vi "WaitUntilVIDoneRunning.vi"(8 "error in (no error)":errorcluster, 11 "UI_Interaction_Manager in":refnum<class "UI_Interaction_Manager.lvclass">) -> (0 "error out":errorcluster, 3 "UI_Interaction_Manager out":refnum<class "UI_Interaction_Manager.lvclass">)   [LabVIEW 2011, in "UI_Interaction_Manager.lvclass"]
uses:
  UI_Interaction_Manager.lvclass
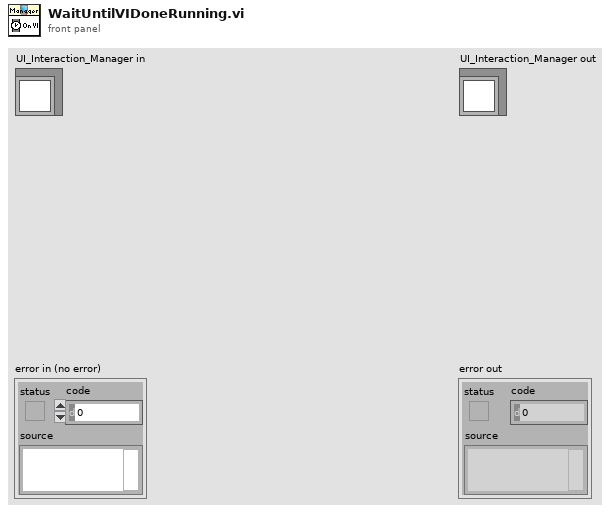
[diagram p1: front panel]
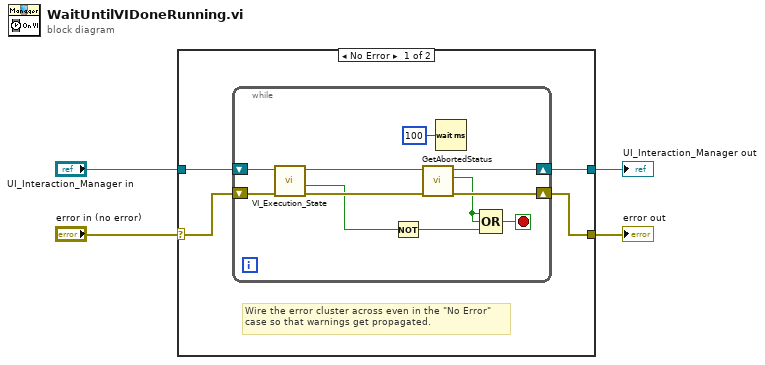
[diagram p0: block diagram]
diagram:
  n1 = case shown="No Error" "error in (no error)" {
    selector: "error in (no error)" -> [w8 w21]
    tunnel: [w7 w21] -> w3
    tunnel: [w5 w20] -> w2
    tunnel: "UI_Interaction_Manager in" -> [w6 w20]
    frame No Error {
      # "Wire the error cluster across even in the \"No Error\"\ncase so that warnings get propagated."
      n2 = while {
        shift-right: [w17] -> w5
        shift-left: w6 -> [w9]
        shift-right: [w15] -> w7
        shift-left: w8 -> [w13]
        stop <- w16 stop-if-true
        n3 = call "VI_Execution_State.vi"("error in (no error)"=w13, "UI_Interaction_Manager in"=w9) -> ("error out"=w18:errorcluster, "Running?"=w11:bool, "UI_Interaction_Manager out"=w19:refnum<class "UI_Interaction_Manager.lvclass">)  [unwired: 6 in, 1 out]
        n4 = Not(x=w11) -> (.not. x?=w12:bool)
        n5 = call "GetAbortedStatus.vi"("error in (no error)"=w18, "UI_Interaction_Manager in"=w19) -> ("error out"=w15:errorcluster, "Aborted?"=w14:bool, "UI_Interaction_Manager out"=w17:refnum<class "UI_Interaction_Manager.lvclass">)  [unwired: 7 in]
        n6 = Wait (ms)(milliseconds to wait=u32 100) -> ()  [unwired: 1 out]
        n7 = Compound Arithmetic op=OR(w14, w14, w12) -> (w16:bool)
      }
    }
    frame Error {
    }
  }
  "error out" <- w3
  "UI_Interaction_Manager out" <- w2
